vi "Estou_no_server.vi"() -> (2 "Estou no serve?":bool)   [LabVIEW 2019]
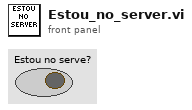
[diagram p1: front panel]
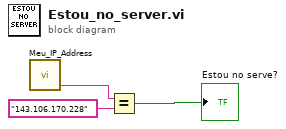
[diagram p0: block diagram]
diagram:
  n1 = call "Meu_IP_Address.vi"() -> ("Meu IP"=w3:string)  [unwired: 4 in, 1 out]
  n2 = Equal?(x=w3, y="143.106.170.228") -> (x = y?=→"Estou no serve?":bool)
